vi "Lowpass (FPGA).vi"   [LabVIEW 2011]
uses:
  Instance           1 22Saved   Lowpass (FPGA) .vi
  <vilib>/rvi/eio/common/nirviEmuTemplateMethod_errors.vi
  <vilib>/rvi/interface/RandomDataEmulation/nirviRandomDataFPGAFIFO.vi
  <vilib>/rvi/interface/RandomDataEmulation/niFpgaRandomDataHandleErrors.vi
  <vilib>/eio/EIONode/EIONode.xnode
  <vilib>/rvi/DataTransferAndStorage/Container/XNode/niFpgaContainer.xnode
  <vilib>/rvi/interface/RandomDataEmulation/nirviRandomDataFpgaReadWriteTemplate.vi
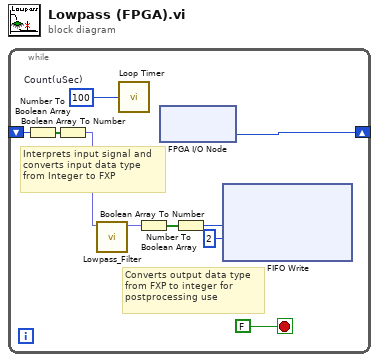
[diagram p0: block diagram]
diagram:
  n1 = while {
    shift-right: [w7] -> _
    shift-left: _ -> [w6]
    stop <- FALSE stop-if-true
    w8 = u16 100  # Count(uSec)
    # "Converts output data type\nfrom FXP to integer for\npostprocessing use"
    # "Interprets input signal and \nconverts input data type\nfrom Integer to FXP"
    n2 = Number To Boolean Array(number=w6) -> (Boolean array=w5:bool[])
    n3 = Boolean Array To Number(Boolean array=w5) -> (number=w4:fxp<+/-,16,1>)
    n4 = call "Lowpass_Filter.vi"("input data"=w4) -> ("output data"=w3:fxp<+/-,32,4>)  [unwired: 1 in, 9 out]
    n5 = call "Loop Timer"("Count(uSec)"=w8) -> ()  [unwired: 1 out]
    n6 = Number To Boolean Array(number=w3) -> (Boolean array=w2:bool[])
    n7 = xnode "FPGA I/O Node"() -> ("AI0"=w7:i16)  [unwired: 1 in, 1 out]
    n8 = Boolean Array To Number(Boolean array=w2) -> (number=w1:i32)
    n9 = xnode ("FIFO Write")("Element"=w1, "Timeout"=2) -> ()  [unwired: 1 in, 2 out]
  }
